vi "Upload_To_ADAM_Server.vi"(0 "Channel Names":string[](array[string]), 1 "Averaging Period (s)":dbl=1.0, 2 "Channel Values":dbl[](array[numeric]), 3 "Shift In":dbl[](array[numeric])) -> (5 "Shift Out":dbl[](array[numeric]))   [LabVIEW 2010]
uses:
  ADAM Controls/Update_scan_value.ctl
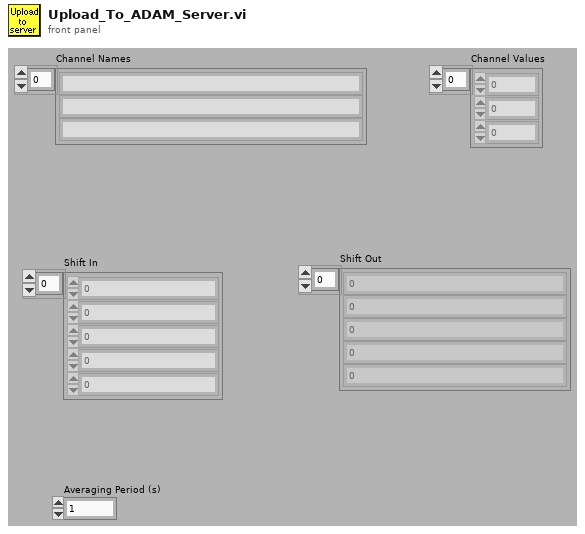
[diagram p1: front panel]
types:
  T1 = typedef "Update_scan_value.ctl" = cluster{"Channel Name":string, "New Value":dbl}
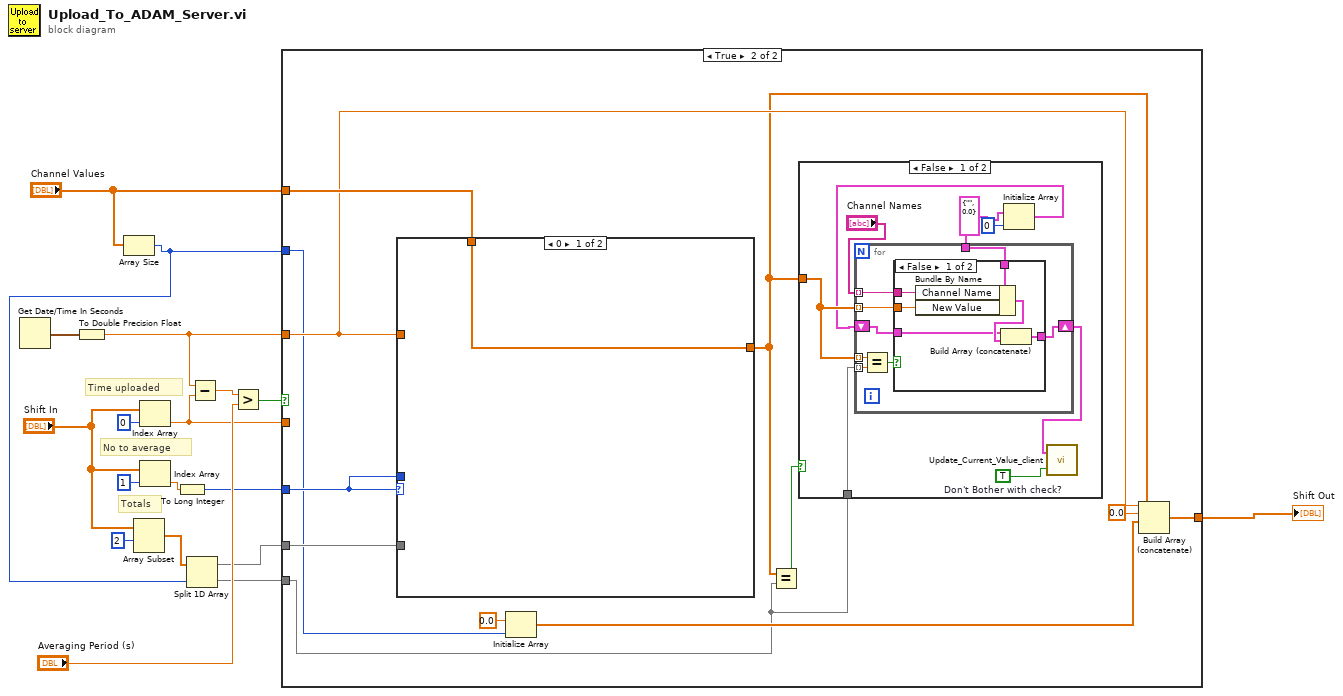
[diagram p0: block diagram]
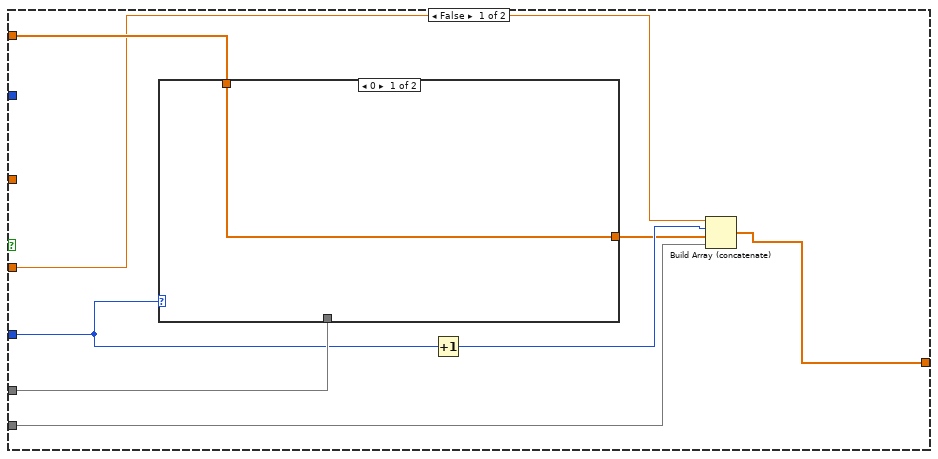
[diagram p2: hidden frame]
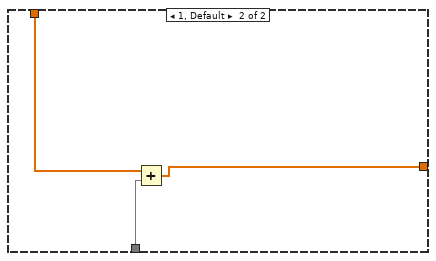
[diagram p3: hidden frame]
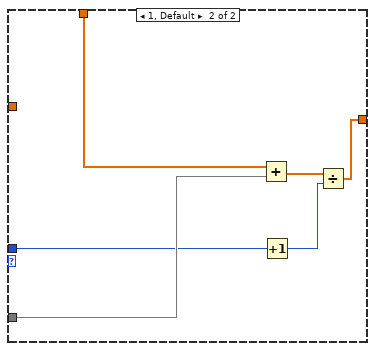
[diagram p6: hidden frame]
diagram:
  # "Totals"
  # "No to average"
  # "Time uploaded"
  n1 = Get Date/Time In Seconds() -> (seconds since 1Jan1904=w17:timestamp)
  n2 = To Double Precision Float(number=w17) -> (double precision float=w8:dbl)
  n3 = Array Size(array="Channel Values") -> (size(s)=w3:i32)
  n4 = Array Subset(array="Shift In", index=2) -> (w4:dbl[])  [unwired: 1 in]
  n5 = Index Array(array="Shift In", index=0) -> (element=w6:dbl)
  n6 = Index Array(array="Shift In", index=1) -> (element=w10:dbl)
  n7 = To Long Integer(number=w10) -> (32bit integer=w9:i32)
  n8 = Split 1D Array(array=w4, index=w3) -> (first subarray=w2:dbl[], second subarray=w1:dbl[])
  n9 = Subtract(x=w8, y=w6) -> (x-y=w16:dbl)
  n10 = Greater?(x=w16, y="Averaging Period (s)") -> (0:w14:bool)
  n11 = case shown="True" w14 {
    tunnel: "Channel Values" -> [w26 w42]
    tunnel: w2 -> [w25 w37]
    tunnel: w9 -> [w23 w41]
    tunnel: w8 -> [_ w40]
    tunnel: [w20 w38] -> w7
    tunnel: w6 -> [w24 _]
    tunnel: w3 -> [_ w34]
    tunnel: w1 -> [w19 w31]
    frame False {
      n12 = case shown="0" w23 {
        tunnel: w26 -> [w27 w30]
        tunnel: w25 -> [_ w29]
        tunnel: [w27 w28] -> w21
        frame 0 {
        }
        frame 1, Default {
          n13 = Add(x=w30, y=w29) -> (x+y=w28:dbl[])
        }
      }
      n14 = Increment(x=w23) -> (x+1=w22:i32)
      n15 = Build Array (concatenate)(w24, w22, w21, w19) -> (w20:dbl[])
    }
    frame True {
      n16 = case shown="0" w41 {
        tunnel: w40 -> [_ _]
        tunnel: w37 -> [_ w71]
        tunnel: w42 -> [w66 w72]
        tunnel: w41 -> [_ w70]
        tunnel: [w66 w67] -> w33
        frame 0 {
        }
        frame 1, Default {
          n17 = Add(x=w72, y=w71) -> (x+y=w69:dbl[])
          n18 = Increment(x=w70) -> (x+1=w68:i32)
          n19 = Divide(x=w69, y=w68) -> (x/y=w67:dbl[])
        }
      }
      n20 = Initialize Array(0.0 ("element"), w34) -> (w35:dbl[])
      n21 = Equal?(x=w33, y=w31) -> (x = y?=w32:bool)
      n22 = case shown="False" w32 {
        tunnel: w33 -> [w49 _]
        tunnel: w31 -> [w48 _]
        frame False {
          w50 = TRUE  # Don't Bother with check?
          w47 = T1 {"Channel Name"="", "New Value"=0.0} ("Update Scan Value Cluster")
          n23 = Initialize Array(w47, 0 ("dimension size")) -> (w45:T1[])
          n24 = for {
            tunnel: w47 -> [w58]
            tunnel: "Channel Names" -> [w57] mode=indexing
            tunnel: w49 -> [w56] mode=indexing
            shift-right: [w51] -> w44
            shift-left: w45 -> [w52]
            tunnel: w49 -> [w55] mode=indexing
            tunnel: w48 -> [w54] mode=indexing
            n25 = Equal?(x=w55, y=w54) -> (x = y?=w53:bool)
            n26 = case shown="False" w53 {
              tunnel: w58 -> [w64 _]
              tunnel: w57 -> [w63 _]
              tunnel: w56 -> [w62 _]
              tunnel: w52 -> [w60 w65]
              tunnel: [w59 w65] -> w51
              frame False {
                n27 = Bundle By Name(cluster=w64, "Channel Name"=w63, "New Value"=w62) -> (w61:T1)
                n28 = Build Array (concatenate)(w60, w61) -> (w59:T1[])
              }
              frame True {
              }
            }
          }
          n29 = call "Update_Current_Value_client.vi"("Don't Bother with check?"=w50, "Update array in"=w44) -> ()
        }
        frame True {
        }
      }
      n30 = Build Array (concatenate)(w40, 0.0 ("element"), w35, w33) -> (w38:dbl[])
    }
  }
  "Shift Out" <- w7
